vi "Source Group Type 2 Text.vi"(10 "Source":T1) -> (3 "String":string)   [LabVIEW 2013]
uses:
  Names/Source Group Type.ctl
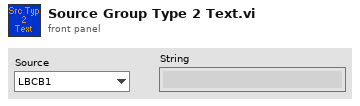
[diagram p1: front panel]
types:
  T1 = typedef "Source Group Type.ctl" = enum16{"LBCB1", "LBCB2", "Consolidated", "External"}
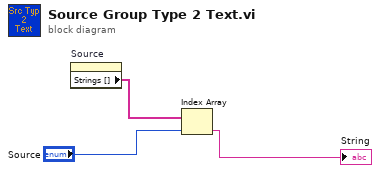
[diagram p0: block diagram]
diagram:
  n1 = property on="Source" class="Enum (strict)"() -> ("Strings []"=w1:string[])  [unwired: 2 in, 2 out]
  n2 = Index Array(array=w1, index="Source") -> (element=→"String":string)
